vi "Read Output value.vi"(8 "error in (no error)":errorcluster, 11 "Set Output Msg in":refnum<class "Set Output Msg.lvclass">) -> (0 "error out":errorcluster, 2 "Output Value.lvclass":refnum<class "Output Value.lvclass">, 3 "Set Output Msg out":refnum<class "Set Output Msg.lvclass">)   [LabVIEW 2016, in "Set Output Msg.lvclass"]
uses:
  Set Output Msg.lvclass
  NHMFL_Core/Libraries/Utilities/Output Value/Output Value.lvclass
  Set Output Msg.lvclass/Set Output Msg.ctl
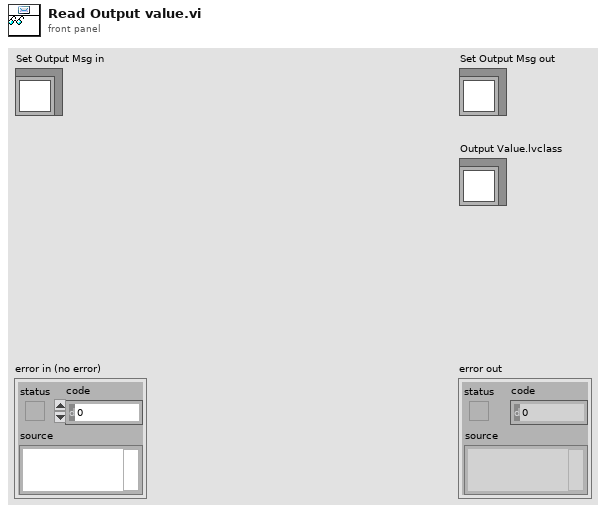
[diagram p1: front panel]
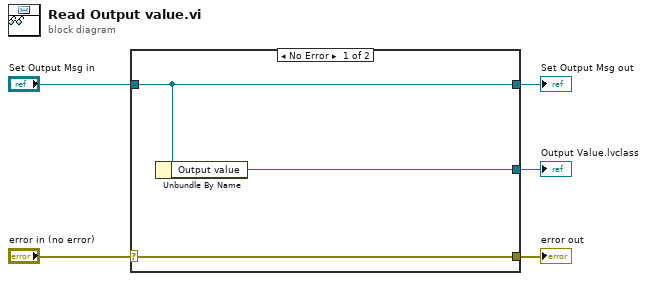
[diagram p0: block diagram]
diagram:
  n1 = case shown="No Error" "error in (no error)" {
    selector: "error in (no error)" -> [w8 w9]
    tunnel: [w8 w9] -> w4
    tunnel: [w7 w10] -> w2
    tunnel: "Set Output Msg in" -> [w7 w10]
    tunnel: [w6 _] -> w1
    frame No Error {
      n2 = Unbundle By Name(w7) -> ("Output value"=w6:refnum<class "Output Value.lvclass">)
    }
    frame Error {
    }
  }
  "error out" <- w4
  "Set Output Msg out" <- w2
  "Output Value.lvclass" <- w1
